vi "Async Actor.vi"(7 "Actor in":refnum<class "Actor.lvclass">, 10 "Spawn":refnum<class "Spawn.lvclass">) -> (0 "Error out":errorcluster, 5 "Actor out":refnum<class "Actor.lvclass">)   [LabVIEW 2025, in "jettl.lvlib" / "Core Actor.lvlib" / "Core Actor.lvclass"]
uses:
  Core Actor.lvclass
  Actor/Actor.lvclass
  Spawn/Spawn/Spawn.lvclass
  Refs/Refs.lvclass
  Core Actor.lvclass/Core Actor.ctl
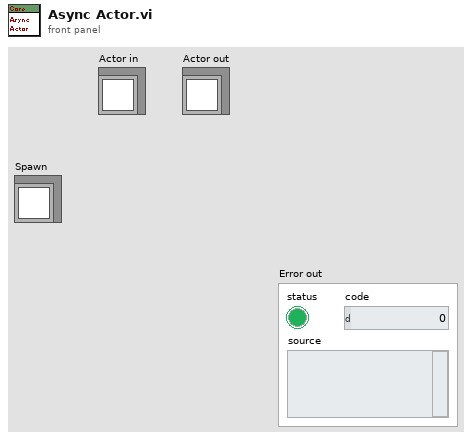
[diagram p1: front panel]
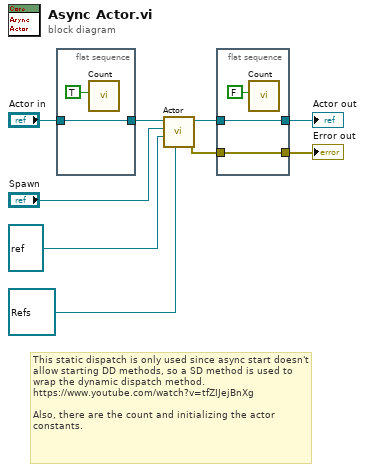
[diagram p0: block diagram]
diagram:
  # "This static dispatch is only used since async start doesn't allow starting DD methods, so a SD method is used to wrap the dynamic dispatch method.\nhttps://www.youtube.com/watch?v=tfZIJejBnXg\n\nAlso, there are the count and initializing the actor constants."
  n1 = flat-sequence {
    tunnel: [w10] -> w6
    tunnel: "Actor in" -> [w10]
    frame #0 {
      n2 = call "Count.vi"("Increment?"=TRUE) -> ()  [unwired: 11 in]
    }
  }
  n3 = call-dynamic "Actor.vi"("Refs"=refnum<class "Refs.lvclass"> refnum, "Actor Ref"=refnum<vi> refnum, "Spawn"="Spawn", "Actor in"=w6) -> ("Error out"=w7:errorcluster, "Actor out"=w8:refnum<class "Actor.lvclass">)  [unwired: 6 in]
  n4 = flat-sequence {
    tunnel: [w13] -> w9
    tunnel: w7 -> [w13]
    tunnel: [w12] -> w5
    tunnel: w8 -> [w12]
    frame #0 {
      n5 = call "Count.vi"("Increment?"=FALSE) -> ()  [unwired: 11 in]
    }
  }
  "Error out" <- w9
  "Actor out" <- w5
